vi "Configure Multi Eval Meas Power Spectrum Density Limit.vi"(6 "Relative (0)":dbl format="%^.3e", 7 "Absolute (0)":dbl format="%^.3e", 8 "error in (no error)":errorcluster, 9 "Spectrum Limits (On)":bool=TRUE, 10 "Instance (1)":i32=1, 11 "VISA resource name":refnum<visa-resource-name>) -> (0 "error out":errorcluster, 3 "VISA resource name out":refnum<visa-resource-name>)   [LabVIEW 2020, in "Rohde&Schwarz CMP LR WPAN Measurement.lvlib"]
doc: "Defines upper limits of power spectrum density for the absolute power and for the power relative to the reference power.\n\nOrder of parameters:\n<PSDAbsolute>\n<PSDRelative>\n<PSDEnabled> - Disable or enable limit check.\n\nAttribute:\n-\n\nRemote-control command:\nCONFigure:WPAN:MEAS<i>:MEValuation:LIMit:SPECtrum"
uses:
  <instrlib>/Rohde&Schwarz CMP LR WPAN Measurement/Rohde&Schwarz CMP LR WPAN Measurement.lvlib
  <instrlib>/Rohde&Schwarz CMP LR WPAN Measurement/Private/rsidr_core.llb/rsidr_core.lvlib
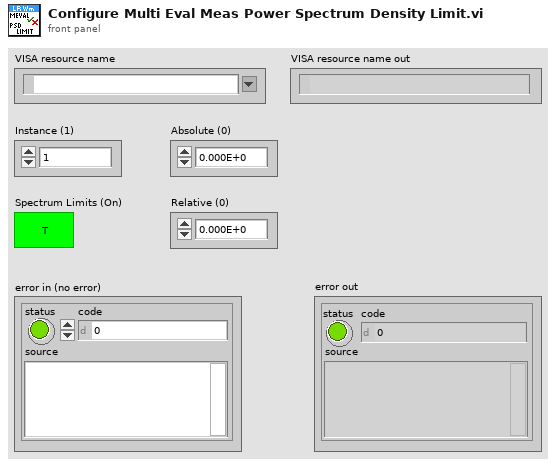
[diagram p1: front panel]
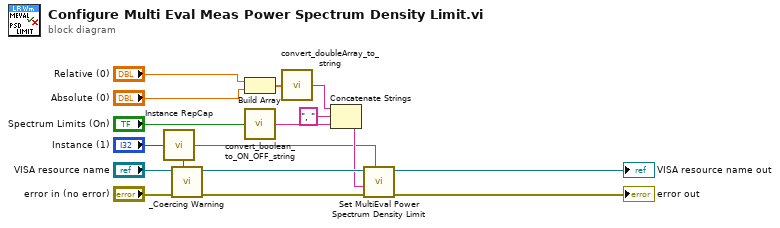
[diagram p0: block diagram]
diagram:
  n1 = call <instrlib>:"Instance RepCap.vi"("Instance In"="Instance (1)") -> ("In Range?"=w17:bool, "RepCap Identifier Out"=w6:string)  [unwired: 1 in]
  n2 = call <instrlib>:"_Coercing Warning.vi"("In Range?"=w17, "error in (no error)"="error in (no error)", "VISA resource name"="VISA resource name") -> ("error out"=w12:errorcluster, "VISA resource name out"=w11:refnum<visa-resource-name>)  [unwired: 7 in]
  n3 = Build Array("Relative (0)", "Absolute (0)") -> (w16:dbl[])
  n4 = call <instrlib>:"convert_boolean_to_ON_OFF_string.vi"("boolean value in"="Spectrum Limits (On)") -> ("string value out"=w15:string)  [unwired: 4 in]
  n5 = call <instrlib>:"convert_doubleArray_to_string.vi"("double array in"=w16) -> ("string out"=w4:string)  [unwired: 4 in]
  n6 = Concatenate Strings(w4, ", " ("string"), w15) -> (w8:string)
  n7 = call "Set MultiEval Power Spectrum Density Limit"("Repeated Capabilities"=w6, "error in (no error)"=w12, "MultiEval Power Spectrum Density Limit ()"=w8, "instrument handle"=w11) -> ("error out"=→"error out":errorcluster, "instrument handle out"=→"VISA resource name out":refnum<visa-resource-name>)  [unwired: 6 in]
